vi "合法性检查.vi"(3 "error in (no error)":errorcluster, 4 "字符串库":string[](array[string]), 5 "被检查字符串":string) -> (0 "error out":errorcluster, 2 "输入有效":bool)   [LabVIEW 2013]
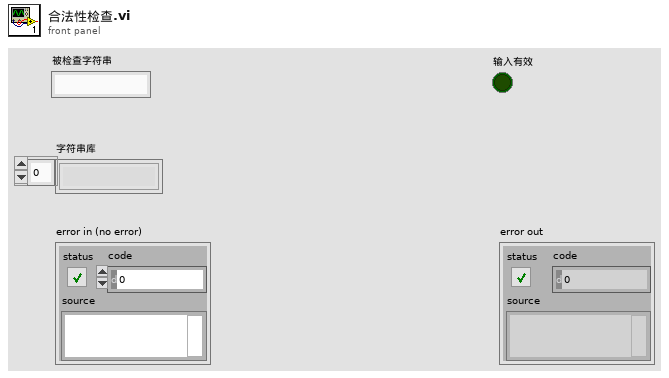
[diagram p1: front panel]
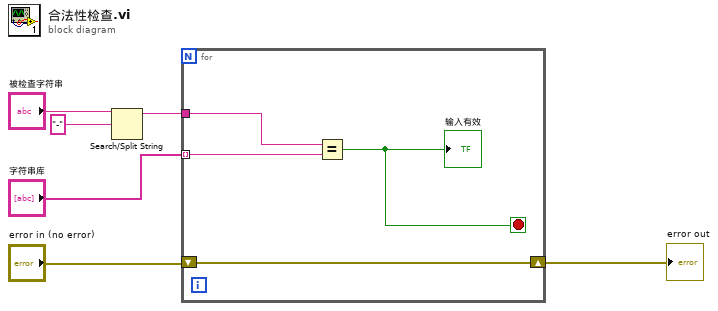
[diagram p0: block diagram]
diagram:
  n1 = Search/Split String(string="被检查字符串", search string/char (-)="-") -> (substring before match=w2:string)  [unwired: 1 in, 2 out]
  n2 = for {
    tunnel: "字符串库" -> [w10] mode=indexing
    shift-right: [w9] -> w4
    shift-left: "error in (no error)" -> [w9]
    tunnel: w2 -> [w7]
    stop <- w8 stop-if-true
    n3 = Equal?(x=w7, y=w10) -> (x = y?=w8:bool)
    "输入有效" <- w8
  }
  "error out" <- w4
